vi "ShowConsole.vi"(8 "error in (no error)":errorcluster, 11 "reference in":refnum<class "Console.lvclass">) -> (0 "error out":errorcluster, 3 "reference out":refnum<class "Console.lvclass">)   [LabVIEW 2018, in "Console.lvclass"]
uses:
  Console.lvclass
panel:
  out "console":string
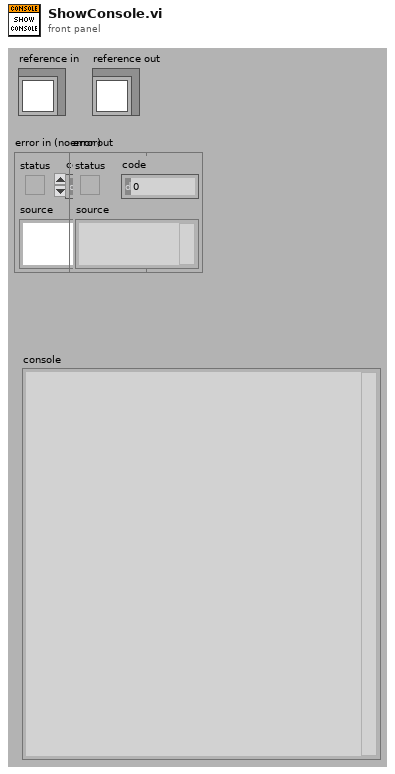
[diagram p1: front panel]
types:
  T1 = enum32{"Invalid", "Standard", "Closed", "Hidden", "Minimized", "Maximized"}
  T2 = typedef "Console.lvclass/ObjectAttributes.ctl" = cluster{"data":string, "count":dbl, "ConsoleRef":refnum<vi>}
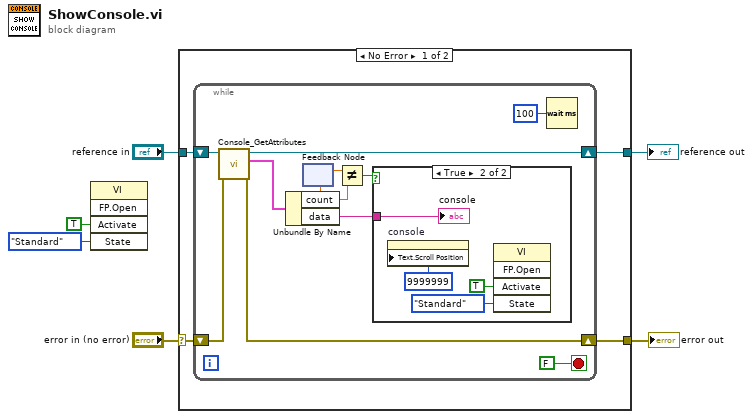
[diagram p0: block diagram]
diagram:
  n1 = invoke class="VI" method="FP.Open"("Activate"=TRUE ("Activate?"), "State"=T1."Standard") -> ()  [unwired: 3 in, 5 out]
  n2 = case shown="No Error" "error in (no error)" {
    selector: "error in (no error)" -> [w10 w27]
    tunnel: [w9 w27] -> w5
    tunnel: [w7 w26] -> w3
    tunnel: "reference in" -> [w8 w26]
    frame No Error {
      n3 = while {
        shift-right: [w19] -> w9
        shift-left: w10 -> [w21]
        shift-right: [w17] -> w7
        shift-left: w8 -> [w18]
        stop <- FALSE stop-if-true
        n4 = call "Console_GetAttributes.vi"("error in (no error)"=w21, "reference in"=w18) -> ("error out"=w19:errorcluster, "Data"=w20:T2, "reference out"=w17:refnum<class "Console.lvclass">)  [unwired: 6 in, 1 out]
        n5 = Unbundle By Name(w20) -> ("count"=w12:dbl, "data"=w16:string)
        n6 = feedback-in #1(w12) -> ()
        n7 = feedback #1() -> (w13:dbl)  [unwired: 1 in]
        n8 = Not Equal?(x=w13, y=w12) -> (x != y?=w11:bool)
        n9 = case shown="True" w11 {
          tunnel: w16 -> [_ w25]
          frame False {
          }
          frame True {
            n10 = property on="console" class="Str"("Text.Scroll Position"=u32 9999999) -> ()  [unwired: 2 in, 2 out]
            n11 = invoke class="VI" method="FP.Open"("Activate"=TRUE ("Activate?"), "State"=T1."Standard") -> ()  [unwired: 3 in, 5 out]
            "console" <- w25
          }
        }
        n12 = Wait (ms)(milliseconds to wait=u32 100) -> ()  [unwired: 1 out]
      }
    }
    frame Error {
    }
  }
  "error out" <- w5
  "reference out" <- w3
